vi "get_nx_juese.vi"(8 "data_name":string, 11 "state":dbl) -> (0 "nx_juese":string, 3 "error":errorcluster caption="error out 4")   [LabVIEW 2017, in "Lib_code.lvlib"]
uses:
  Lib_code.lvlib
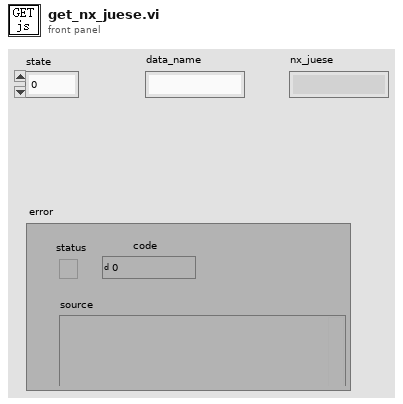
[diagram p1: front panel]
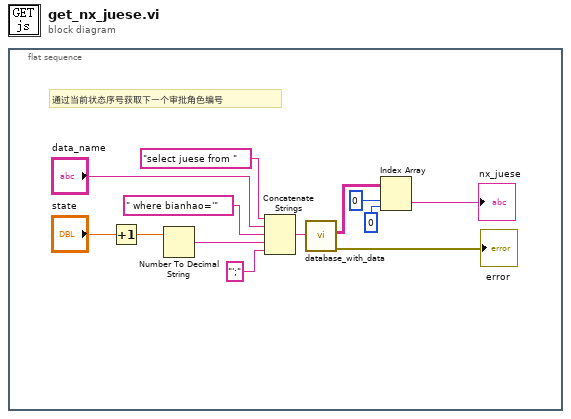
[diagram p0: block diagram]
diagram:
  n1 = flat-sequence {
    frame #0 {
      # "通过当前状态序号获取下一个审批角色编号"
      n2 = Increment(x="state") -> (x+1=w11:dbl)
      n3 = Number To Decimal String(number=w11) -> (decimal integer string=w10:string)  [unwired: 1 in]
      n4 = Concatenate Strings("select juese from " ("Command Text"), "data_name", " where bianhao='" ("字符串"), w10, "';" ("字符串")) -> (w5:string)
      n5 = call "database_with_data.vi"("input"=w5) -> ("error"=→"error":errorcluster, "Data"=w4:string[][])  [unwired: 9 in]
      n6 = Index Array(array=w4, index (row)=0 ("索引 (行)"), index (col)=0 ("禁用的索引 (列)")) -> (element=→"nx_juese":string)
    }
  }
